vi "read json file.vi"(11 "File Path":path) -> (0 "error out":errorcluster, 3 "Data out":T1)   [LabVIEW 2020, in "Template.lvlib" / "Template.lvclass"]
uses:
  Template.lvclass
  typedefs/actor configuration.ctl
  typedefs/shared actor configuration.ctl
  typedefs/resource config/device configuration cluster.ctl
  typedefs/resource config/single resource cluster.ctl
  3c470e21-1639-4616-9875-34d8c0f16db8.vi
  465192f6-cf10-4ed9-8c5f-bfc9042509a2.vi
  <vilib>/JDP Science/JSONtext/JSON text to Variant.vi
  <vilib>/JDP Science/JSONtext/Variant to JSON Text.vi
  <vilib>/JDP Science/JSONtext/LVClass Serializer/JSONtext LVClass Serializer.lvclass
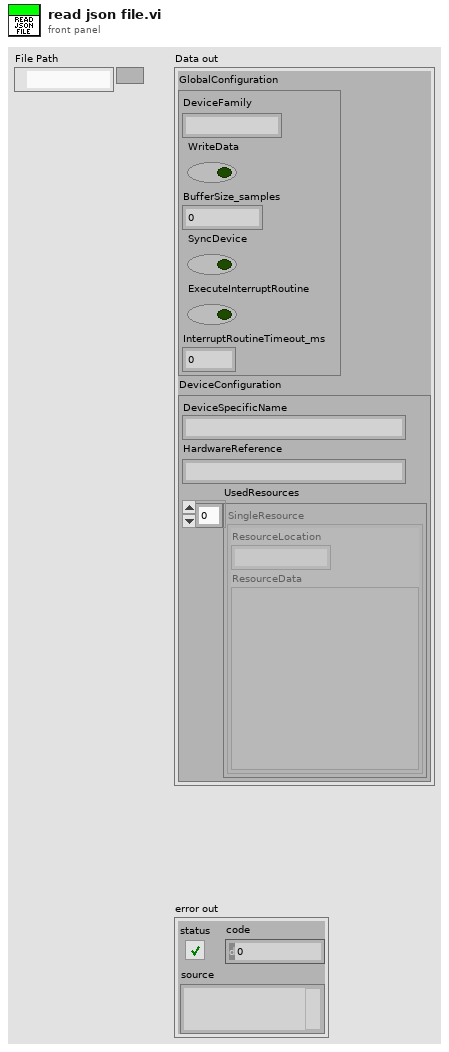
[diagram p1: front panel]
types:
  T1 = typedef "Template.lvlib/Template.lvclass/actor configuration.ctl" = cluster{"GlobalConfiguration":T2, "DeviceConfiguration":T3}
  T2 = typedef "Template.lvlib/Template.lvclass/shared actor configuration.ctl" = cluster{"DeviceFamily":string, "WriteData":bool, "BufferSize_samples":i32, "SyncDevice":bool, "ExecuteInterruptRoutine":bool, "InterruptRoutineTimeout_ms":i32}
  T3 = typedef "Template.lvlib/Template.lvclass/device configuration cluster.ctl" = cluster{"DeviceSpecificName":string, "HardwareReference":string, "UsedResources":T4[]}
  T4 = typedef "Template.lvlib/Template.lvclass/single resource cluster.ctl" = cluster{"ResourceLocation":string, "ResourceData":variant}
  T5 = enum16{"open", "replace", "create", "open or create", "replace or create", "replace or create with confirmation"}
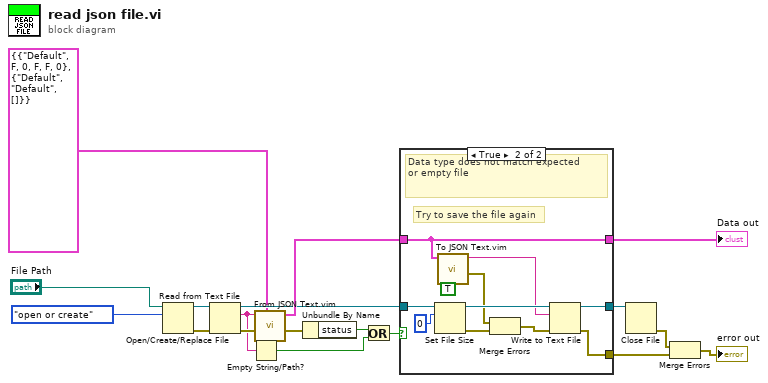
[diagram p0: block diagram]
diagram:
  n1 = Open/Create/Replace File(file path (use dialog)="File Path", operation (0:open)=T5."open or create") -> (refnum out=w8:refnum<file>, error out=w9:errorcluster)  [unwired: 4 in, 1 out]
  n2 = Read from Text File(file (use dialog)=w8, error in=w9) -> (refnum out=w12:refnum<file>, text=w5:string, error out=w10:errorcluster)  [unwired: 2 in, 1 out]
  n3 = Empty String/Path?(string/path=w5) -> (empty?=w1:bool)
  n4 = call "From JSON Text.vim"("Data Type and Default Value"=T1 {"GlobalConfiguration"={"DeviceFamily"="Default", "WriteData"=FALSE, "BufferSize_samples"=0, "SyncDevice"=FALSE, "ExecuteInterruptRoutine"=FALSE, "InterruptRoutineTimeout_ms"=0}, "DeviceConfiguration"={"DeviceSpecificName"="Default", "HardwareReference"="Default", "UsedResources"=[]}} ("ActorConfiguration"), "error in (no error)"=w10, "JSON"=w5) -> ("error out"=w4:errorcluster, "Data out"=w13:T1)  [unwired: 7 in]
  n5 = Unbundle By Name(w4) -> ("status"=w3:bool)
  n6 = Or(x=w3, y=w1) -> (x .or. y?=w2:bool)
  n7 = case shown="True" w2 {
    tunnel: w12 -> [w20 w31]
    tunnel: w13 -> [w19 w21]
    tunnel: [w20 w24] -> w14
    tunnel: [_ w23] -> w15
    tunnel: [w19 w21] -> w18
    frame False {
      # "Normal operation."
    }
    frame True {
      # "Try to save the file again"
      # "Data type does not match expected\nor empty file"
      n8 = Set File Size(6:i64 0 ("size (in bytes)"), 7:w31) -> (0:w28:errorcluster, 3:w29:refnum<file>)  [unwired: 1 in]
      n9 = call "To JSON Text.vim"("Pretty Print?"=TRUE, "Anything"=w21) -> ("error out"=w25:errorcluster, "<JSON>"=w27:string)  [unwired: 8 in]
      n10 = Merge Errors(w25, w28) -> (w26:errorcluster)
      n11 = Write to Text File(file (use dialog)=w29, text=w27, error in=w26) -> (refnum out=w24:refnum<file>, error out=w23:errorcluster)  [unwired: 1 in, 1 out]
    }
  }
  "Data out" <- w18
  n12 = Close File(refnum=w14) -> (error out=w17:errorcluster)  [unwired: 1 in, 1 out]
  n13 = Merge Errors(w17, w15) -> (→"error out":errorcluster)
